vi "GetCellStrColor.vi"(7 "Color":u32, 8 "error in (no error)":errorcluster, 10 "Hdr Name":T1, 11 "Voltage in":refnum<class "Voltage.lvclass">) -> (0 "error out":errorcluster, 1 "Cell String":string, 2 "Cell Color":u32, 3 "Voltage out":refnum<class "Voltage.lvclass">)   [LabVIEW 2018, in "Measurement Channels.lvlib" / "Voltage.lvclass"]
uses:
  Voltage.lvclass
  Common/Controls/HeaderNames.ctl
  SubVIs Table/Custom Ctls Table/ge_ColType.ctl
  Voltage.lvclass/Voltage.ctl
  Class Channel/Channel.lvclass
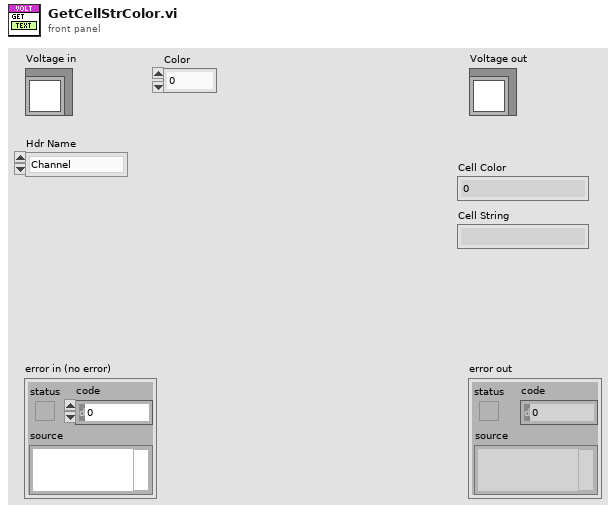
[diagram p1: front panel]
types:
  T1 = typedef "HeaderNames.ctl" = enum16{"Channel", "Device", "Spacer", "Description", "MB", "Range", "Terminal", "Coupling", "Thresh (V)", "Pulse/Rev", "Slope", "Min EU", "Min RPM", "mV/EU", "Iex", "Temp Units", "Type", "CJC Src", "CJC Val", "Ro", "Wire Cfg", "Strain Mode", "Vex", "Bridge Type", "GF", "Gauge Res", "Poisson", "Lead Res", "Init Strain", "GAF", "Scale", "Offset", "Unit (EU)", "dB?", "dB Ref", "Cal Mag", "Cal Units", "Max Temp", "Min Temp", "Max Strain", "Min Strain"}
  T2 = typedef "ge_ColType.ctl" = enum16{"Volts", "Amps", "Ohms", "TermCfg", "WireCfg", "Coup", "Slope", "Iex", "CalUnits", "ThrmUnits", "ThrmType", "CJCSrc", "BrdgType", "Strn Mode", "RTDType"}
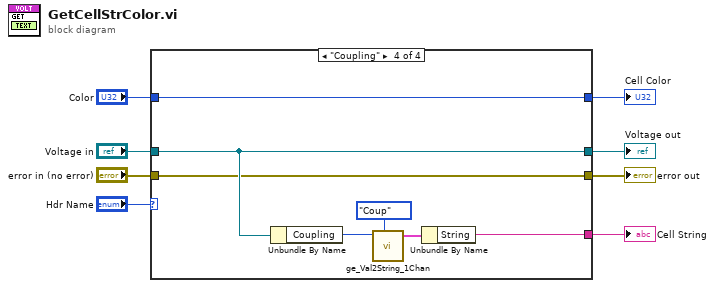
[diagram p0: block diagram]
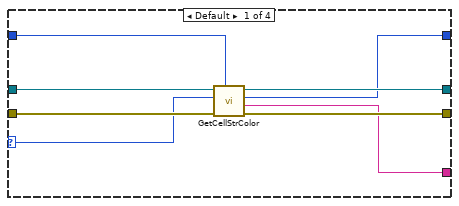
[diagram p2: hidden frame]
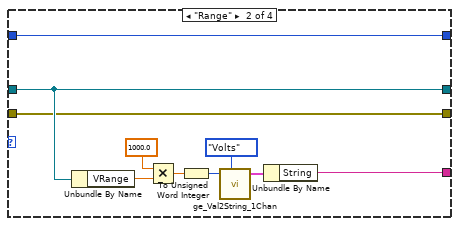
[diagram p3: hidden frame]
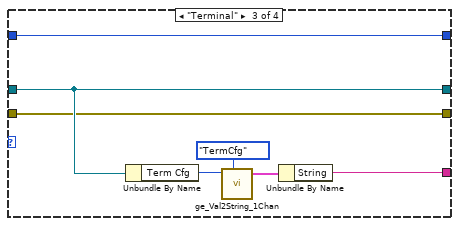
[diagram p4: hidden frame]
diagram:
  n1 = case shown="\"Coupling\"" "Hdr Name" {
    selector: "Hdr Name" -> [w12 _ _ _]
    tunnel: "Voltage in" -> [w16 w18 w28 w35]
    tunnel: [w9 w20 w31 w38] -> w6
    tunnel: [w10 w19 w29 w36] -> w7
    tunnel: "Color" -> [w11 w19 w29 w36]
    tunnel: [w15 w18 w28 w35] -> w5
    tunnel: "error in (no error)" -> [w14 w17 w27 w34]
    tunnel: [w13 w17 w27 w34] -> w1
    frame Default {
      n2 = call-parent "GetCellStrColor.vi"("Color"=w11, "error in (no error)"=w14, "Hdr Name"=w12, "Channel in"=w16) -> ("error out"=w13:errorcluster, "Cell String"=w9:string, "Cell Color"=w10:u32, "Channel out"=w15:refnum<class "Voltage.lvclass">)  [unwired: 4 in]
    }
    frame "Range" {
      n3 = Unbundle By Name(w18) -> ("VRange"=w23:dbl)
      n4 = Multiply(x=1000.0, y=w23) -> (x*y=w22:dbl)
      n5 = To Unsigned Word Integer(number=w22) -> (unsigned 16bit integer=w26:u16)
      n6 = call "ge_Val2String_1Chan.vi"("Value"=w26, "ColType"=ge_ColType."Volts") -> ("String and Val"=w24:cluster{"String":string, "Value":u16})  [unwired: 5 in]
      n7 = Unbundle By Name(w24) -> ("String"=w20:string)
    }
    frame "Terminal" {
      n8 = Unbundle By Name(w28) -> ("Term Cfg"=w30:u16)
      n9 = call "ge_Val2String_1Chan.vi"("Value"=w30, "ColType"=ge_ColType."TermCfg") -> ("String and Val"=w32:cluster{"String":string, "Value":u16})  [unwired: 5 in]
      n10 = Unbundle By Name(w32) -> ("String"=w31:string)
    }
    frame "Coupling" {
      n11 = Unbundle By Name(w35) -> ("Coupling"=w37:u16)
      n12 = call "ge_Val2String_1Chan.vi"("Value"=w37, "ColType"=ge_ColType."Coup") -> ("String and Val"=w39:cluster{"String":string, "Value":u16})  [unwired: 5 in]
      n13 = Unbundle By Name(w39) -> ("String"=w38:string)
    }
  }
  "error out" <- w1
  "Voltage out" <- w5
  "Cell String" <- w6
  "Cell Color" <- w7
